vi "potencia a corriente(1).vi"(1 "Max current A":dbl, 2 "Potencia":dbl) -> (0 "Corriente":dbl)   [LabVIEW 2016]
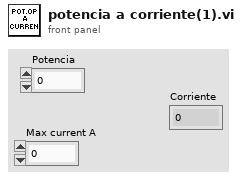
[diagram p1: front panel]
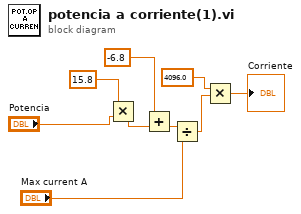
[diagram p0: block diagram]
diagram:
  n1 = Multiply(x=15.8, y="Potencia") -> (x*y=w7:dbl)
  n2 = Add(x=-6.8, y=w7) -> (x+y=w5:dbl)
  n3 = Divide(x=w5, y="Max current A") -> (x/y=w8:dbl)
  n4 = Multiply(x=4096.0, y=w8) -> (x*y=→"Corriente":dbl)
